vi "Send Log Packet.vi"(8 "error in (no error)":errorcluster, 10 "Log Data":T1={"Time"=timestamp(0 s since 1904-01-01), "Level"=enum."INFO", "Logger"="", "Message"="", "Arguments"=[]} {"Time" format="%<%x %.3X>T"}, 11 "Log Sinks in":refnum<class "Log Sinks.lvclass">) -> (0 "error out":errorcluster, 3 "Log Sinks out":refnum<class "Log Sinks.lvclass">)   [LabVIEW 2019, in "TSC Event Logger.lvlib" / "Log Sinks.lvclass"]
doc: "encrypt the log data (if applicable) and send to the sink\n\n<b>Code Developed By:</b>\nTechnology Service Corporation\nBloomington, IN 47403\nwww.tsc.com/atcs\n\nDeveloper:\nDaniel Coons"
uses:
  Log Sinks.lvclass
  Log Data.ctl
  Log/Event Level.ctl
  Log Sinks.lvclass/Log Sinks.ctl
  Encryption/Encryption.lvclass
  TSC Event Logger.lvlib
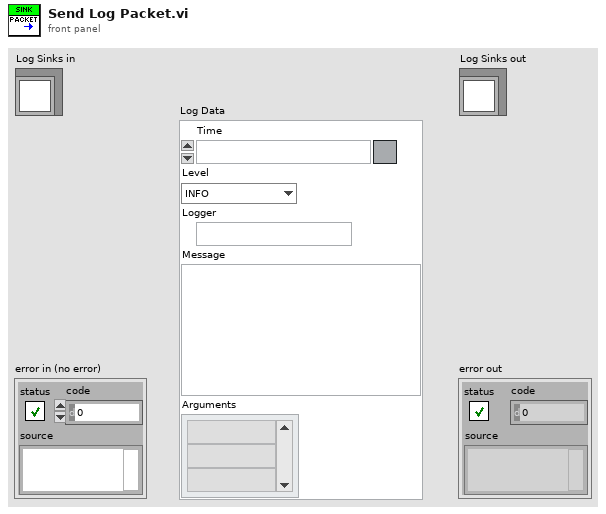
[diagram p1: front panel]
types:
  T1 = typedef "TSC Event Logger.lvlib/Log Data.ctl" = cluster{"Time":timestamp, "Level":T2, "Logger":string, "Message":string, "Arguments":string[]}
  T2 = typedef "TSC Event Logger.lvlib/Event Level.ctl" = enum16{"OFF", "TRACE", "DEBUG", "INFO", "WARN", "ERROR", "FATAL"}
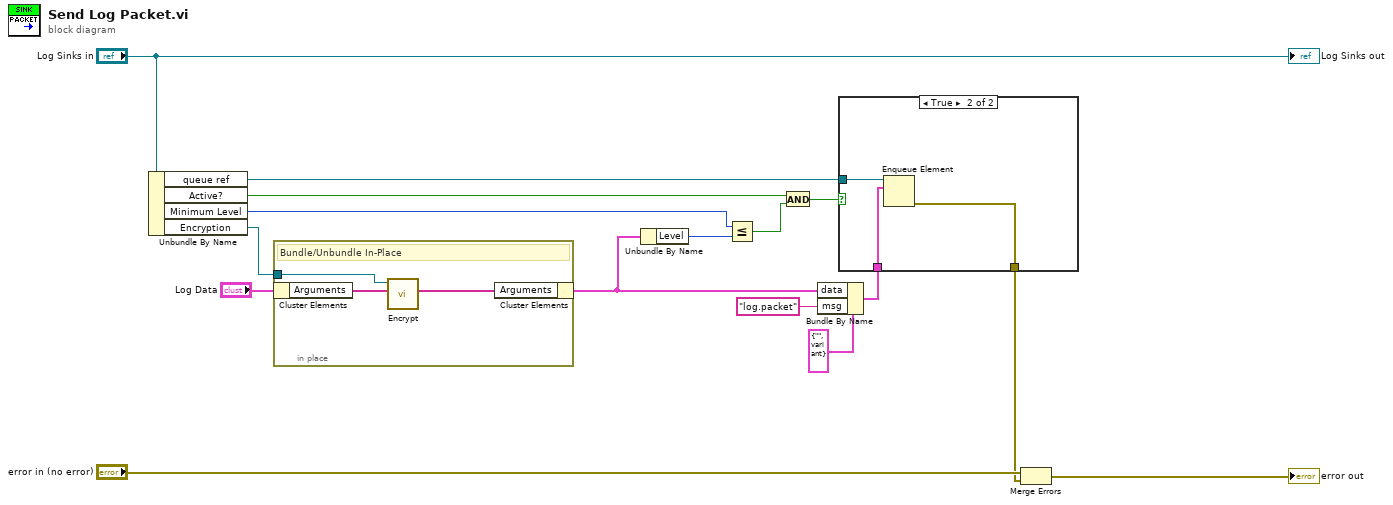
[diagram p0: block diagram]
diagram:
  n1 = Unbundle By Name("Log Sinks in") -> ("queue ref"=w14:refnum<queue>, "Active?"=w6:bool, "Minimum Level"=w9:T2, "Encryption"=w1:refnum<class "Encryption.lvclass">)
  n2 = in-place {
    in-place-border: w1 -> [w17]
    # "Bundle/Unbundle In-Place"
    n3 = in-place-cluster #1("Log Data") -> ("Arguments"=w19:string[])
    n4 = call-dynamic "Encrypt.vi"("Arguments"=w19, "Encryption in"=w17) -> ("Encrypted Arguments"=w18:string[])  [unwired: 7 in, 2 out]
    n5 = in-place-cluster #1("Arguments"=w18) -> (w2:T1)
  }
  n6 = Unbundle By Name(w2) -> ("Level"=w8:T2)
  n7 = Less Or Equal?(x=w9, y=w8) -> (x <= y?=w7:bool)
  n8 = And(x=w6, y=w7) -> (x .and. y?=w5:bool)
  n9 = Bundle By Name(cluster=cluster{"msg":string, "data":variant} {"msg"="", "data"=variant} ("element"), "data"=w2, "msg"="log.packet") -> (w12:cluster{"msg":string, "data":variant})
  n10 = case shown="True" w5 {
    tunnel: w14 -> [_ w22]
    tunnel: w12 -> [_ w21]
    tunnel: [_ w20] -> w10
    frame False {
    }
    frame True {
      n11 = Enqueue Element(queue=w22, element=w21) -> (error out=w20:errorcluster)  [unwired: 2 in, 2 out]
    }
  }
  n12 = Merge Errors("error in (no error)", w10) -> (→"error out":errorcluster)
  "Log Sinks out" <- "Log Sinks in"
